vi "CloseIMAQdxCamera.vi"   [LabVIEW 2015]
uses:
  <vilib>/userdefined/High Color/IMAQdx.ctl
  <vilib>/vision/driver/NI_Vision_Acquisition_Software.lvlib
types:
  T1 = typedef "IMAQdx.ctl" = refnum<k21>
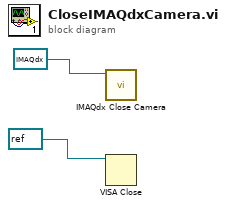
[diagram p0: block diagram]
diagram:
  n1 = call <vilib>:"IMAQdx Close Camera.vi"("Session In"=T1 refnum) -> ()  [unwired: 10 in, 1 out]
  n2 = VISA Close(VISA resource name=refnum<visa-resource-name> refnum ("VISA资源名称")) -> ()  [unwired: 1 in, 1 out]
